vi "Analisis de Img.vi"(4 "error in":errorcluster, 10 "File Path in":path, 11 "Número de elementos":i32) -> (0 "error out":errorcluster, 1 "Image Out 2":T1, 2 "concatenated string":string, 3 "Refnum out":T1, 5 "path":path, 6 "Medición":string)   [LabVIEW 2017]
uses:
  <vilib>/vision/Image Controls.llb/IMAQ Image.ctl
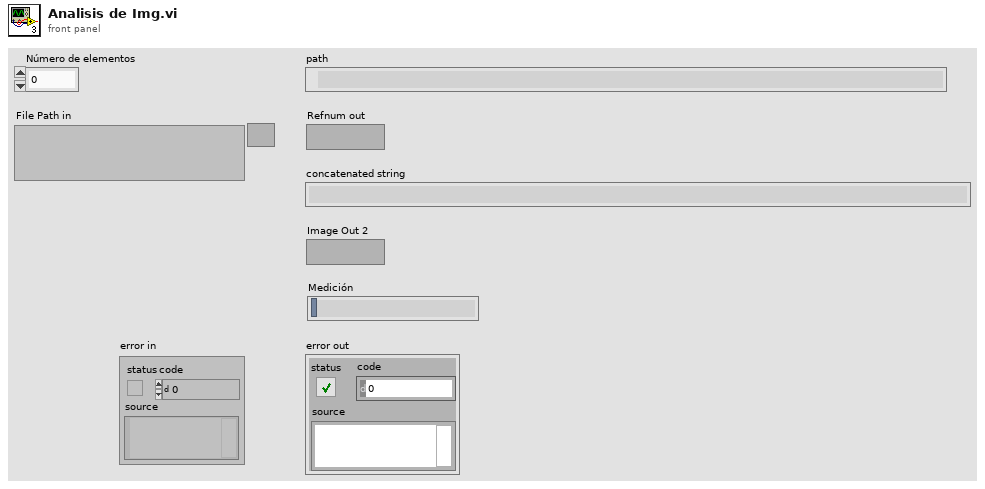
[diagram p1: front panel]
types:
  T1 = typedef "IMAQ Image.ctl" = refnum<image>
  T2 = typedef "Image Type" = u32
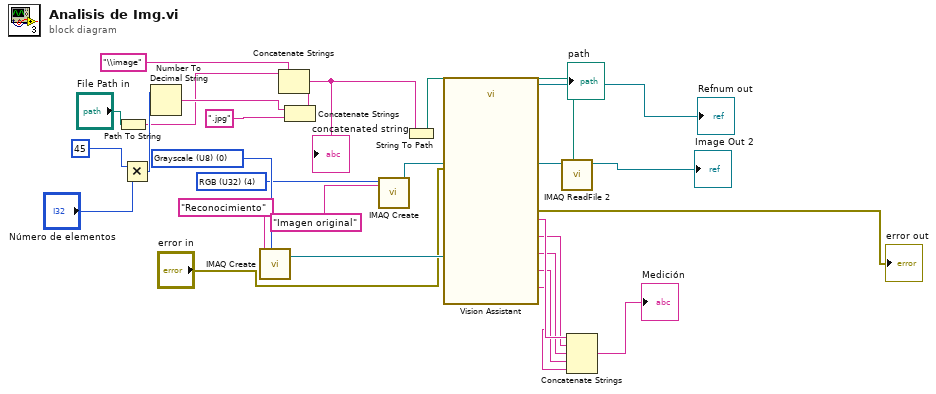
[diagram p0: block diagram]
diagram:
  w15 = T2 0 items=["Grayscale (U8)", "Grayscale (I16)", "Grayscale (SGL)", "Complex (CSG)", "RGB (U32)", "HSL (U32)", "RGB (U64)", "Grayscale (U16)"] ("Image Type")
  w14 = T2 4 items=["Grayscale (U8)", "Grayscale (I16)", "Grayscale (SGL)", "Complex (CSG)", "RGB (U32)", "HSL (U32)", "RGB (U64)", "Grayscale (U16)"] ("Image Type")
  n1 = Path To String(path="File Path in") -> (string=w17:string)
  n2 = Multiply(x=45, y="Número de elementos") -> (x*y=w20:i32)
  n3 = Number To Decimal String(number=w20) -> (decimal integer string=w23:string)  [unwired: 1 in]
  n4 = call "IMAQ Create"("Image Name"="Reconocimiento", "Image Type"=w15) -> ("New Image"=w13:T1)  [unwired: 3 in, 1 out]
  n5 = Concatenate Strings(w23, ".jpg" ("string")) -> (w25:string)
  n6 = Concatenate Strings(w17, "\\image", w25) -> (w21:string)
  "concatenated string" <- w21
  n7 = call "IMAQ Create"("Image Name"="Imagen original", "Image Type"=w14) -> ("New Image"=w10:T1)  [unwired: 3 in, 1 out]
  n8 = String To Path(string=w21) -> (path=w22:path)
  "path" <- w22
  n9 = call "IMAQ ReadFile 2"("File Path"=w22, "Image"=w10) -> ("Image Out"=w11:T1)  [unwired: 5 in, 4 out]
  "Image Out 2" <- w11
  n10 = call "Vision Assistant"("Image In"=w11, "Image Dst"=w13, "error in"="error in") -> ("Image Out"=→"Refnum out":T1, "String (OCR/OCV 3)"=w8:string, "String (OCR/OCV 4)"=w7:string, "String (OCR/OCV 5)"=w6:string, "String (OCR/OCV 6)"=w5:string, "String (OCR/OCV 7)"=w4:string, "error out"=→"error out":errorcluster)  [unwired: 18 in]
  n11 = Concatenate Strings(w8, w7, w6, w5, w4) -> (→"Medición":string)
